vi "Teleop.vi"(10 "Match Info":T1={"Autonomous Elapsed Seconds"=0.0, "TeleOp Elapsed Seconds"=0.0, "Disabled Elapsed Seconds"=0.0, "Visited Autonomous"=FALSE, "Visited TeleOp"=FALSE, "Visited Disabled"=FALSE, "Autonomous Settings"={"Autonomous Style"=enum."Independent", "VI Refnum"=refnum}}, 11 "Call Context":T2) -> ()   [LabVIEW 2013]
doc: "This VI is called for each TeleOp packet received from the DS where the robot is not disabled. It is often used to read from the joysticks and update I/O or to update setpoints for timed control loops. It should complete and return within 20 milliseconds or it may miss DS packets."
uses:
  <vilib>/Rock Robotics/WPI/DriverStation/WPI_DriverStationDerivedRobotMode.ctl
  <vilib>/Rock Robotics/WPI/DriverStation/WPI_DriverStationMatch Info.ctl
  <vilib>/Rock Robotics/WPI/Solenoid/WPI_SolenoidValue.ctl
  Robot Global Data.vi
  <vilib>/Rock Robotics/WPI/Joystick/WPI_JoystickGetSetRefNum.vi
  <vilib>/Rock Robotics/WPI/Solenoid/WPI_SolenoidSetEnum.vi
  <vilib>/Rock Robotics/WPI/RobotDrive/WPI_RobotDriveGetSetRefNum.vi
panel:
  out "Distance (in.) Back":dbl
  out "Distance (ft.) Back":dbl
  out "Distance (in.)":dbl
  out "Distance (ft.)":dbl
  out "Distance Right":dbl
  out "Distance Left":dbl
  out "Numeric 1":dbl(slide) scale=0.0..100.0
  out "Boolean 2":bool
  out "Boolean 1":bool
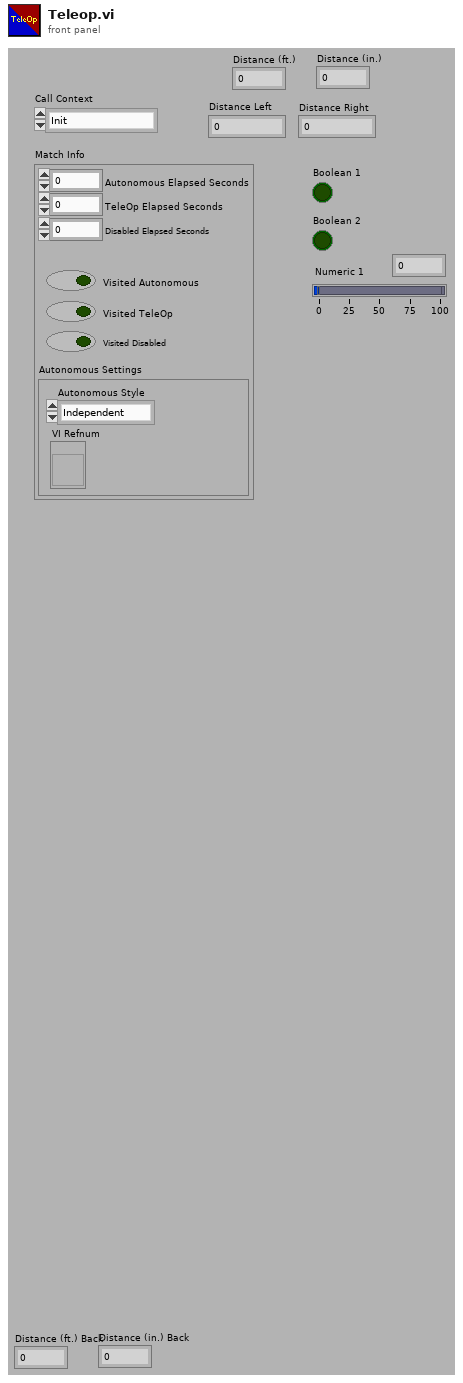
[diagram p1: front panel]
types:
  T1 = typedef "WPI_DriverStationMatch Info.ctl" = cluster{"Autonomous Elapsed Seconds":dbl, "TeleOp Elapsed Seconds":dbl, "Disabled Elapsed Seconds":dbl, "Visited Autonomous":bool, "Visited TeleOp":bool, "Visited Disabled":bool, "Autonomous Settings":cluster{"Autonomous Style":enum16{"Iterative", "Independent"}, "VI Refnum":refnum<vi>}}
  T2 = typedef "WPI_DriverStationDerivedRobotMode.ctl" = enum16{"Init", "Execute", "Stop"}
  T3 = enum8{"Backward Spin WOT", "Forward Spin WOT", "Disengage WOT", "Engage WOT", "Kiddy Control", "Fire"}[]
  T4 = typedef "WPI_EncoderDevRef.ctl" = cluster{"DevStatus":errorcluster, "EncoderIndex":T5, "CounterIndex":T6, "DistancePerCount":dbl, "Decoding Type":T7}
  T5 = typedef "FPGA_EncoderIdx.ctl" = enum8{"Enc 0", "Enc 1", "Enc 2", "Enc 3", "Invalid"}
  T6 = typedef "FPGA_CounterCtrSystemIndex.ctl" = enum8{"Ctr 0", "Ctr 1", "Ctr 2", "Ctr 3", "Ctr 4", "Ctr 5", "Ctr 6", "Ctr 7", "Invalid"}
  T7 = typedef "WPI_EncoderType.ctl" = enum16{"1x", "2x", "4x"}
  T8 = typedef "WPI_AnalogChannelDevRef.ctl" = cluster{"DevStatus":errorcluster, "Analog Module":T9, "Analog Channel":T10}
  T9 = typedef "FPGA_TypedefAnalogModule.ctl" = enum16{"Analog Module 1", "Analog Module 2"}
  T10 = typedef "FPGA_AIChannel.ctl" = enum8{"AI 1", "AI 2", "AI 3", "AI 4", "AI 5", "AI 6", "AI 7", "AI 8", "Invalid"}
  T11 = typedef "WPI_JoystickDevRef.ctl" = cluster{"Device":T12}
  T12 = typedef "WPI_JoystickDeviceEnum.ctl" = enum16{"USB 1", "USB 2", "USB 3", "USB 4", "Kinect 1", "Kinect 2"}
  T13 = typedef "WPI_JoystickButtonState.ctl" = cluster{"Button 1":bool, "Button 2":bool, "Button 3":bool, "Button 4":bool, "Button 5":bool, "Button 6":bool, "Button 7":bool, "Button 8":bool, "Button 9":bool, "Button 10":bool, "Button 11":bool, "Button 12":bool}
  T14 = cluster{"axis 1 (x)":dbl, "axis 2 (y)":dbl, "axis 3 (throttle)":dbl, "axis 4":dbl, "axis 5":dbl, "axis 6":dbl}
  T15 = cluster{"Pressed? Array[0]":bool, "Pressed? Array[1]":bool, "Pressed? Array[2]":bool, "Pressed? Array[3]":bool, "Pressed? Array[4]":bool}
  T16 = typedef "WPI_SolenoidValue.ctl" = enum16{"Off", "On", "Forward", "Reverse"}
  T17 = typedef "WPI_SolenoidDevRef.ctl" = cluster{"DevStatus":errorcluster, "Solenoid Module":T18, "Forward Solenoid Channel":T19, "Reverse Solenoid Channel":T19}
  T18 = typedef "FPGA_TypedefSolenoidModule.ctl" = enum16{"Solenoid Module 1", "Solenoid Module 2"}
  T19 = typedef "WPI_SolenoidChannel.ctl" = enum8{"Solenoid 1", "Solenoid 2", "Solenoid 3", "Solenoid 4", "Solenoid 5", "Solenoid 6", "Solenoid 7", "Solenoid 8", "Invalid"}
  T20 = typedef "WPI_RobotDriveDevRef.ctl" = cluster{"DevStatus":errorcluster, "Motors[]":T21[], "Square Inputs":bool, "Max Output":dbl, "Isochronous":bool}
  T21 = typedef "WPI_MotorControlDeviceRef.ctl" = cluster{"DeviceStatus":errorcluster, "Type":enum16{"PWM", "CAN"}, "PWM":cluster{"Digital Module":T22, "PWM Channel":T23, "DeadBand":T24}, "CAN":cluster{"Device Number":u8, "Control Mode":T25, "Semaphore":T26, "Max Vout":dbl}, "Invert":bool, "TransformRef":T27, "InvTransformRef":T27}
  T22 = typedef "FPGA_TypedefDigitalModule.ctl" = enum16{"Digital Module 1", "Digital Module 2"}
  T23 = typedef "FPGA_DIOPWMChannel.ctl" = enum8{"PWM 1", "PWM 2", "PWM 3", "PWM 4", "PWM 5", "PWM 6", "PWM 7", "PWM 8", "PWM 9", "PWM 10", "Invalid"}
  T24 = typedef "WPI_PWMDeadband.ctl" = cluster{"Name":string, "maxPositivePwm":i32, "minPositivePwm":i32, "centerPwm":i32, "maxNegativePwm":i32, "minNegativePwm":i32, "angularRange":u16}
  T25 = typedef "WPI_CANJaguar_ControlMode.ctl" = enum8{"Percent VBus", "Current", "Speed", "Position", "Voltage"}
  T26 = typedef "Semaphore RefNum" = refnum<k1>
  T27 = typedef "WPI_PWMTransform_ConPane.ctl" = refnum<vi>
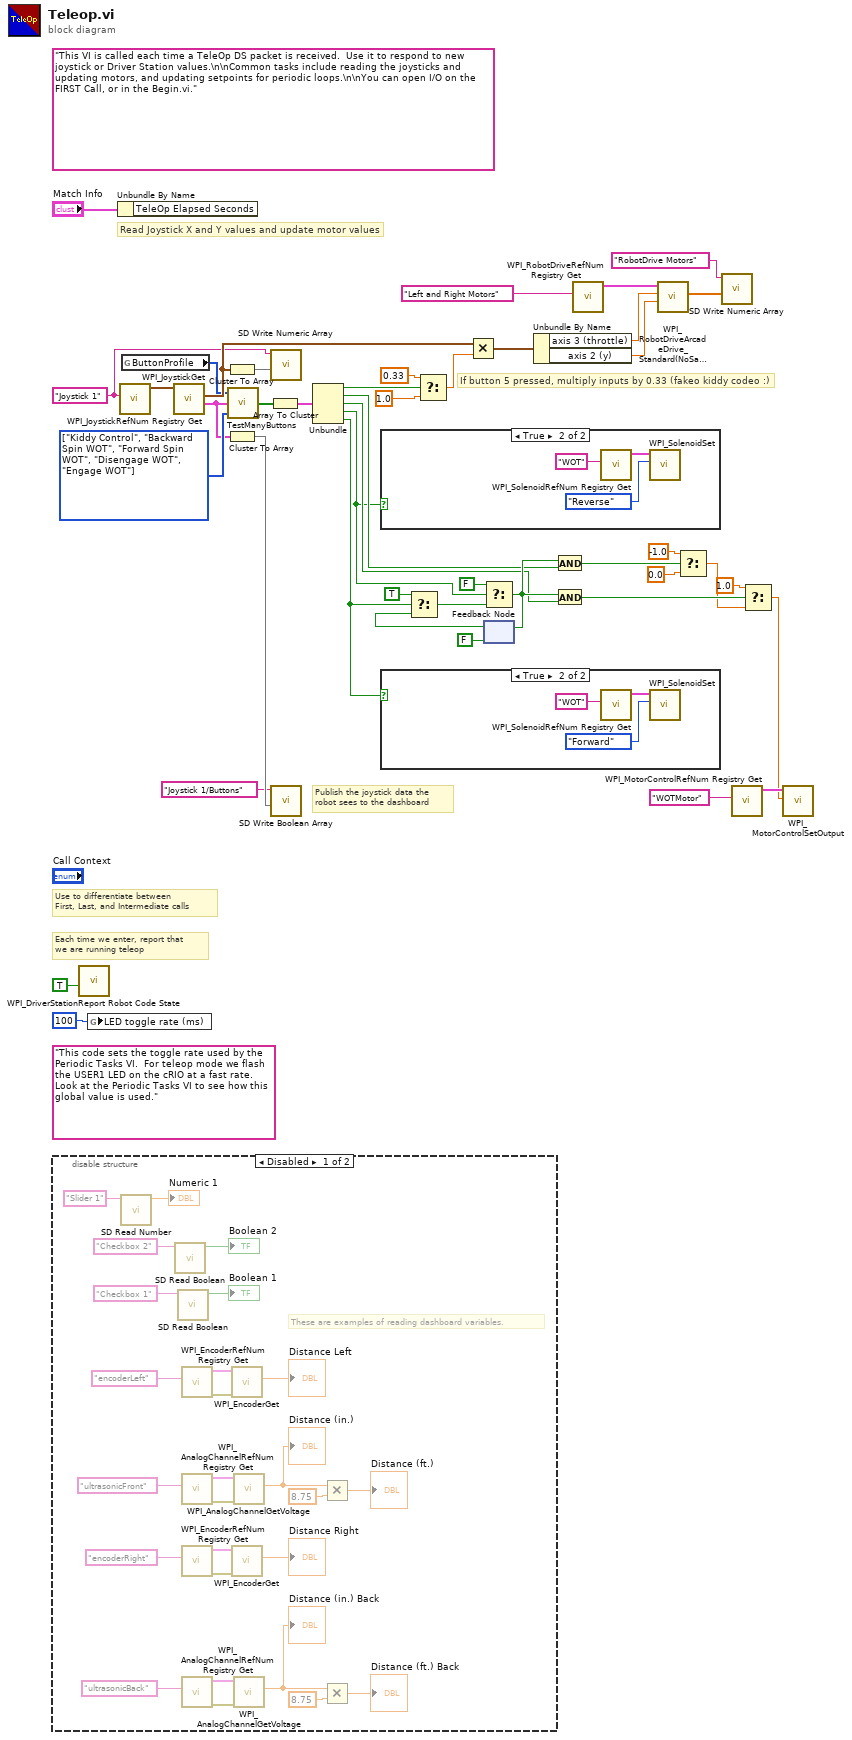
[diagram p0: block diagram]
diagram:
  w10 = T3 [enum."Kiddy Control", enum."Backward Spin WOT", enum."Forward Spin WOT", enum."Disengage WOT", enum."Engage WOT"] items=["Backward Spin WOT", "Forward Spin WOT", "Disengage WOT", "Engage WOT", "Kiddy Control", "Fire"]
  w28 = "Joystick 1" ("Name")
  (unwired) "This code sets the toggle rate used by the Periodic Tasks VI.  For teleop mode we flash the USER1 LED on the cRIO at a fast rate.  Look at the Periodic Tasks VI to see how this global value is used."
  (unwired) "This VI is called each time a TeleOp DS packet is received.  Use it to respond to new joystick or Driver Station values.\n\nCommon tasks include reading the joysticks and updating motors, and updating setpoints for periodic loops.\n\nYou can open I/O on the FIRST Call, or in the Begin.vi."
  # "If button 5 pressed, multiply inputs by 0.33 (fakeo kiddy codeo :)"
  # "Publish the joystick data the\nrobot sees to the dashboard"
  # "Each time we enter, report that\nwe are running teleop"
  # "Use to differentiate between\nFirst, Last, and Intermediate calls"
  # "Read Joystick X and Y values and update motor values"
  n1 = disable-structure shown="Disabled" {
    frame Disabled {
      # "These are examples of reading dashboard variables."
      n2 = call <vilib>:"SD Read Number.vi"("Name"="Slider 1" ("refnum name")) -> ("Numeric"=→"Numeric 1":dbl)  [unwired: 8 in, 2 out]
      n3 = call <vilib>:"SD Read Boolean.vi"("Name"="Checkbox 2" ("refnum name")) -> ("Boolean"=→"Boolean 2":bool)  [unwired: 8 in, 2 out]
      n4 = call <vilib>:"SD Read Boolean.vi"("Name"="Checkbox 1" ("refnum name")) -> ("Boolean"=→"Boolean 1":bool)  [unwired: 8 in, 2 out]
      n5 = call <vilib>:"WPI_EncoderRefNum Registry Get.vi"("refnum name"="encoderLeft") -> ("error out"=w62:errorcluster, "EncoderDevRef"=w63:T4)  [unwired: 9 in]
      n6 = call <vilib>:"WPI_AnalogChannelRefNum Registry Get.vi"("refnum name"="ultrasonicFront") -> ("error out"=w56:errorcluster, "AIDeviceRef"=w55:T8)  [unwired: 9 in]
      n7 = call <vilib>:"WPI_EncoderRefNum Registry Get.vi"("refnum name"="encoderRight") -> ("error out"=w58:errorcluster, "EncoderDevRef"=w59:T4)  [unwired: 9 in]
      n8 = call <vilib>:"WPI_AnalogChannelRefNum Registry Get.vi"("refnum name"="ultrasonicBack") -> ("error out"=w50:errorcluster, "AIDeviceRef"=w49:T8)  [unwired: 9 in]
      n9 = call <vilib>:"WPI_EncoderGet.vi"("error in (no error)"=w62, "EncoderDevRef"=w63) -> ("Distance"=→"Distance Left":dbl)  [unwired: 4 in, 5 out]
      n10 = call <vilib>:"WPI_EncoderGet.vi"("error in (no error)"=w58, "EncoderDevRef"=w59) -> ("Distance"=→"Distance Right":dbl)  [unwired: 4 in, 5 out]
      n11 = call <vilib>:"WPI_AnalogChannelGetVoltage.vi"("error in (no error)"=w56, "AIDeviceRef"=w55) -> ("Voltage"=w51:dbl)  [unwired: 7 in, 2 out]
      "Distance (in.)" <- w51
      n12 = call <vilib>:"WPI_AnalogChannelGetVoltage.vi"("error in (no error)"=w50, "AIDeviceRef"=w49) -> ("Voltage"=w45:dbl)  [unwired: 7 in, 2 out]
      "Distance (in.) Back" <- w45
      n13 = Multiply(x=w51, y=8.75) -> (x*y=→"Distance (ft.)":dbl)
      n14 = Multiply(x=w45, y=8.75) -> (x*y=→"Distance (ft.) Back":dbl)
    }
    frame Enabled {
    }
  }
  n15 = call <vilib>:"WPI_DriverStationReport Robot Code State.vi"("TeleOp"=TRUE ("Autonomous")) -> ()  [unwired: 10 in, 1 out]
  n16 = global write "Robot Global Data.vi" "LED toggle rate (ms)"(u32 100 ("LED ms toggle rate")) -> ()
  n17 = Unbundle By Name("Match Info") -> ()  [unwired: 1 out]
  n18 = call <vilib>:"WPI_JoystickRefNum Registry Get.vi"("refnum name"=w28) -> ("JoystickDevRef"=w39:T11)  [unwired: 1 in, 9 out]
  n19 = global read "Robot Global Data.vi" "ButtonProfile"() -> (w8:u8[])
  n20 = call <vilib>:"WPI_JoystickGet.vi"("JoystickDevRef"=w39) -> ("Buttons"=w9:T13, "Axes"=w33:T14)  [unwired: 1 in, 4 out]
  n21 = Cluster To Array(cluster=w33) -> (array=w36:dbl[])
  n22 = Cluster To Array(cluster=w9) -> (array=w38:bool[])
  n23 = call "TestManyButtons.vi"("Testable Button Array"=w10, "Buttons"=w9, "ButtonProfile"=w8) -> ("Pressed? Array"=w7:bool[])
  n24 = Array To Cluster(array=w7) -> (cluster=w6:T15)
  n25 = call <vilib>:"SD Write Numeric Array.vi"("Numeric Array"=w36, "Name"=w28) -> ()  [unwired: 8 in, 2 out]
  n26 = call <vilib>:"SD Write Boolean Array.vi"("Boolean Array"=w38, "Name"="Joystick 1/Buttons") -> ()  [unwired: 8 in, 2 out]
  n27 = Unbundle(w6) -> ("Pressed? Array[0]"=w5:bool, "Pressed? Array[1]"=w4:bool, "Pressed? Array[2]"=w3:bool, "Pressed? Array[3]"=w2:bool, "Pressed? Array[4]"=w1:bool)
  n28 = case shown="True" w2 {
    frame False {
    }
    frame True {
      n29 = call <vilib>:"WPI_SolenoidRefNum Registry Get.vi"("refnum name"="WOT") -> ("SolenoidDevRef"=w72:T17)  [unwired: 9 in, 1 out]
      n30 = call-poly <vilib>:"WPI_SolenoidSet.vi"("Value"=WPI_SolenoidValue."Reverse" ("t"), "SolenoidDevRef"=w72) -> ()  [unwired: 8 in, 2 out]
    }
  }
  n31 = case shown="True" w1 {
    frame False {
    }
    frame True {
      n32 = call <vilib>:"WPI_SolenoidRefNum Registry Get.vi"("refnum name"="WOT") -> ("SolenoidDevRef"=w75:T17)  [unwired: 9 in, 1 out]
      n33 = call-poly <vilib>:"WPI_SolenoidSet.vi"("Value"=WPI_SolenoidValue."Forward" ("t"), "SolenoidDevRef"=w75) -> ()  [unwired: 8 in, 2 out]
    }
  }
  n34 = Select(t=0.33, s=w5, f=1.0) -> (s? t:f=w32:dbl)
  n35 = Multiply(x=w33, y=w32) -> (x*y=w31:T14)
  n36 = feedback #1(FALSE) -> (w21:bool)
  n37 = Select(t=TRUE, s=w1, f=w21) -> (s? t:f=w23:bool)
  n38 = Select(t=FALSE, s=w2, f=w23) -> (s? t:f=w14:bool)
  n39 = feedback-in #1(w14) -> ()
  n40 = Unbundle By Name(w31) -> ("axis 3 (throttle)"=w27:dbl, "axis 2 (y)"=w26:dbl)
  n41 = And(x=w14, y=w4) -> (x .and. y?=w15:bool)
  n42 = And(x=w14, y=w3) -> (x .and. y?=w19:bool)
  n43 = call <vilib>:"WPI_RobotDriveRefNum Registry Get.vi"("refnum name"="Left and Right Motors") -> ("RobotDriveDevRef"=w40:T20)  [unwired: 1 in, 9 out]
  n44 = call <vilib>:"WPI_RobotDriveArcadeDrive_Standard(NoSaturation).vi"("Y axis value"=w26, "X axis value"=w27, "RobotDriveDevRef"=w40) -> ("Motor Values"=w34:dbl[])  [unwired: 1 in, 7 out]
  n45 = Select(t=-1.0, s=w15, f=0.0 ("t")) -> (s? t:f=w13:dbl)
  n46 = call <vilib>:"SD Write Numeric Array.vi"("Numeric Array"=w34, "Name"="RobotDrive Motors") -> ()  [unwired: 8 in, 2 out]
  n47 = call <vilib>:"WPI_MotorControlRefNum Registry Get.vi"("refnum name"="WOTMotor") -> ("MotorControlDevRef"=w12:T21)  [unwired: 9 in, 1 out]
  n48 = Select(t=1.0, s=w19, f=w13) -> (s? t:f=w11:dbl)
  n49 = call <vilib>:"WPI_MotorControlSetOutput.vi"("Output"=w11, "MotorControlDevRef"=w12) -> ()  [unwired: 7 in, 3 out]
